vi "Read User List.vi"(10 "User List File":path, 11 "User List File Default":path) -> (1 "Array":string[](array[string]), 3 "Path Out":path)   [LabVIEW 2018]
uses:
  <vilib>/Utility/file.llb/Read Delimited Spreadsheet (string).vi
panel:
  # "Outputs"
  # "Inputs"
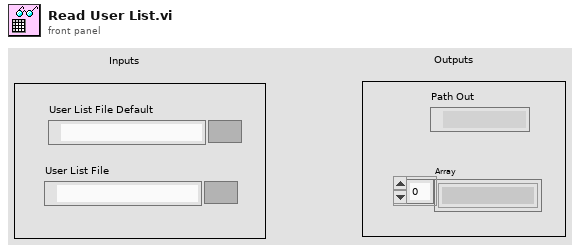
[diagram p1: front panel]
types:
  T1 = enum16{"open", "replace", "create", "open or create", "replace or create", "replace or create with confirmation"}
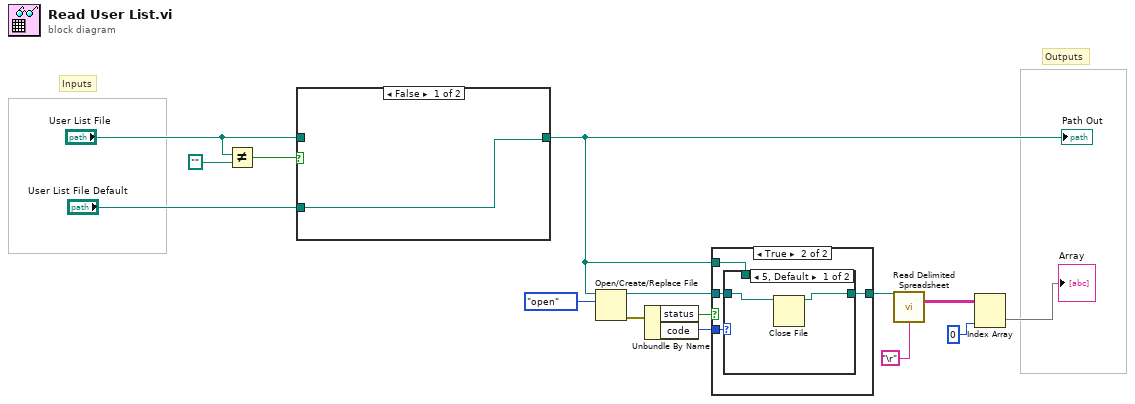
[diagram p0: block diagram]
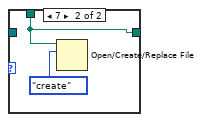
[diagram p3: hidden frame]
diagram:
  # "Inputs"
  # "Outputs"
  n1 = Not Equal?(x="User List File", y=path "") -> (x != y?=w8:bool)
  n2 = case shown="False" w8 {
    tunnel: [w16 w17] -> w1
    tunnel: "User List File" -> [_ w17]
    tunnel: "User List File Default" -> [w16 _]
    frame False {
    }
    frame True {
    }
  }
  "Path Out" <- w1
  n3 = Open/Create/Replace File(file path (use dialog)=w1, operation (0:open)=T1."open") -> (refnum out=w4:refnum<file>, error out=w7:errorcluster)  [unwired: 4 in, 1 out]
  n4 = Unbundle By Name(w7) -> ("status"=w6:bool, "code"=w2:i32)
  n5 = case shown="True" w6 {
    tunnel: w4 -> [_ w21]
    tunnel: [w18 w20] -> w3
    tunnel: w2 -> [_ w22]
    tunnel: w1 -> [w18 w19]
    frame False {
    }
    frame True {
      n6 = case shown="5, Default" w22 {
        tunnel: w21 -> [w24 _]
        tunnel: [w23 w25] -> w20
        tunnel: w19 -> [_ w25]
        frame 5, Default {
          n7 = Close File(refnum=w24) -> (path=w23:path)  [unwired: 1 in, 1 out]
        }
        frame 7 {
          n8 = Open/Create/Replace File(file path (use dialog)=w25, operation (0:open)=T1."create") -> ()  [unwired: 4 in, 3 out]
        }
      }
    }
  }
  n9 = call-poly <vilib>:"Read Delimited Spreadsheet.vi"("file path (dialog if empty)"=w3, "delimiter (\\t)"="\r") -> ("all rows"=w15:string[][])  [unwired: 8 in, 5 out]
  n10 = Index Array(array=w15, index (col)=0) -> (element=→"Array":string[])  [unwired: 1 in]
